vi "Intan_InitSerial.vi"(0 "VISA resource name":refnum<visa-resource-name>="COM1", 2 "InitialChar":string="o", 4 "Nbytes initial response":u32=72) -> (3 "VISA resource name out":refnum<visa-resource-name>, 5 "Text response":string, 6 "error out":errorcluster)   [LabVIEW 2020]
doc: "This VI establishes a serial connection (VISA) with the selected resource and clears the port.\nThe type of resource (USB Serial or Bluetooth) must match the resource name (COM port number). The baud rate is selected automatically based the type of resource. Specifically, the Intan RHD2000 + Teensyduino setup can be configured to run USB serial (9600 baud rate selected, though actual transfer rate is full USB speed); or we can choose to transmit wirelessly using RN-42 Bluetooth module set for 115200 baud.\n\nIn addition, an initial character is set to have Teensy automatically detect which serial port is being used."
uses:
  <vilib>/Instr/_visa.llb/VISA Configure Serial Port (Serial Instr).vi
panel:
  out "return count":u32
  in  "termination char\n(0xA = '\\n' = LF)":u8=4 format="%.0x"
  in  "Enable Termination Char (T)":bool=TRUE
  in  "timeout (2 sec)":u32=4000
  in  "flow control":u16(ring)=2 items=["None"=0, "XON/XOFF"=1, "RTS/CTS"=2, "DTR/DSR"=4]
  in  "stop bits":u16(ring)=10 items=["1.0"=10, "1.5"=15, "2.0"=20]
  in  "parity":u16(ring) items=["None", "Odd", "Even", "Mark", "Space"]
  in  "data bits":u16=8 min=5 max=8 step=1
  out "baud rate":u32=115200
  # "Use this VI to initialize\nserial COM connection\nto Teensy-Intan interface\n\nMake sure to match the port name with the port type"
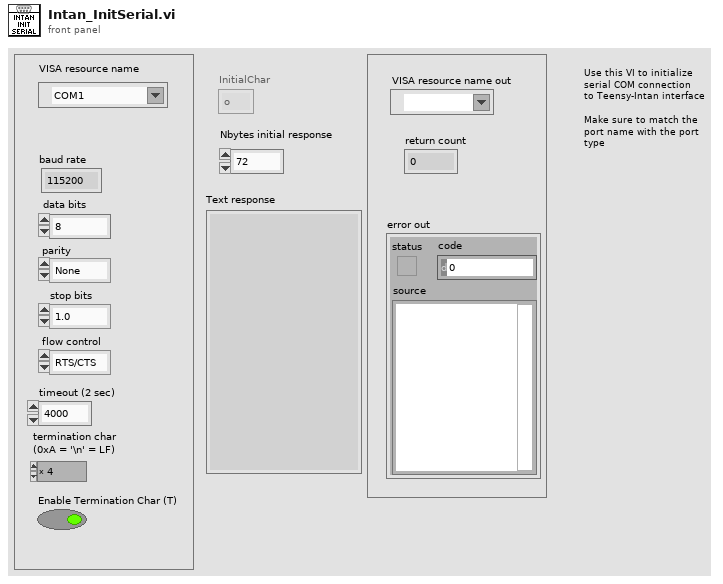
[diagram p1: front panel]
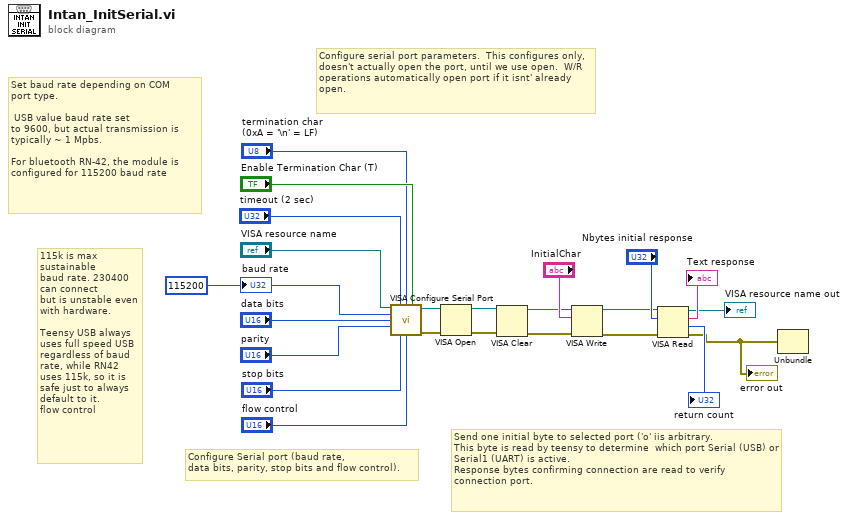
[diagram p0: block diagram]
diagram:
  w2 = u32 115200
  # "115k is max sustainable\nbaud rate. 230400 can connect\nbut is unstable even with hardware.\n\nTeensy USB always uses full speed USB regardless of baud rate, while RN42 uses 115k, so it is safe just to always default to it.\nflow control"
  # "Send one initial byte to selected port ('o' iis arbitrary.\nThis byte is read by teensy to determine  which port Serial (USB) or Serial1 (UART) is active.\nResponse bytes confirming connection are read to verify connection port."
  # "Configure serial port parameters.  This configures only, doesn't actually open the port, until we use open.  W/R operations automatically open port if it isnt' already open."
  # "Set baud rate depending on COM\nport type. \n\n USB value baud rate set \nto 9600, but actual transmission is\ntypically ~ 1 Mpbs.\n\nFor bluetooth RN-42, the module is \nconfigured for 115200 baud rate"
  # "Configure Serial port (baud rate,\ndata bits, parity, stop bits and flow control)."
  n1 = call-poly "VISA Configure Serial Port"("VISA resource name"="VISA resource name", "timeout (10sec)"="timeout (2 sec)", "termination char\n(0xA = '\\n' = LF)"="termination char\n(0xA = '\\n' = LF)", "Enable Termination\nChar (T)"="Enable Termination Char (T)", "baud rate (9600)"=w2, "data bits (8)"="data bits", "parity (0:none)"="parity", "stop bits (10: 1 bit)"="stop bits", "flow control (0:none)"="flow control") -> ("VISA resource name out"=w14:refnum<visa-resource-name>, "error out"=w13:errorcluster)  [unwired: 5 in]
  n2 = VISA Open(error in (no error)=w13, VISA resource name=w14) -> (VISA resource name=w6:refnum<visa-resource-name>, error out=w7:errorcluster)  [unwired: 3 in]
  n3 = VISA Clear(VISA resource name=w6, error in (no error)=w7) -> (VISA resource name out=w5:refnum<visa-resource-name>, error out=w4:errorcluster)
  n4 = VISA Write(VISA resource name=w5, write buffer="InitialChar", error in (no error)=w4) -> (VISA resource name out=w9:refnum<visa-resource-name>, error out=w10:errorcluster)  [unwired: 1 out]
  n5 = VISA Read(VISA resource name=w9, byte count="Nbytes initial response", error in (no error)=w10) -> (VISA resource name out=→"VISA resource name out":refnum<visa-resource-name>, read buffer=→"Text response":string, return count=→"return count":u32, error out=w3:errorcluster)
  "error out" <- w3
  n6 = Unbundle(w3) -> ()  [unwired: 3 out]
  "baud rate" <- w2
